vi "O2 Sensor Simulation.vi"(10 "Lambda":fxp<+,12,3>, 11 "Voltage at Ip in":fxp<+/-,16,5>) -> (0 "Ip":fxp<+/-,32,10>, 3 "Vn Out":fxp<+/-,20,5>)   [LabVIEW 2014]
uses:
  <vilib>/rvi/Analysis/measure/butterworth/XNode/niFpgaButterworthFilter.xnode
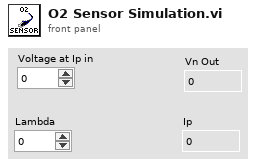
[diagram p1: front panel]
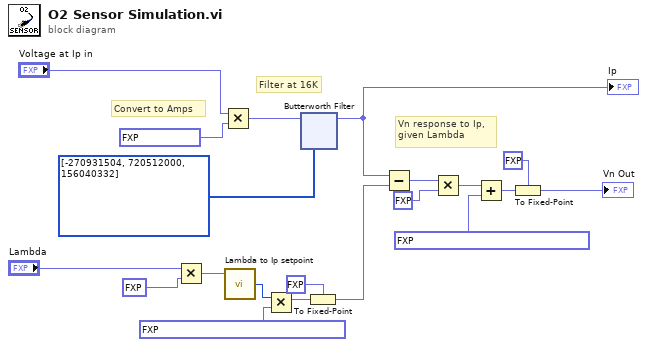
[diagram p0: block diagram]
diagram:
  # "Filter at 16K"
  # "Vn response to Ip, \ngiven Lambda"
  # "Convert to Amps"
  n1 = Multiply(x="Lambda", y=fxp<+,7,7> 100.0) -> (x*y=w17:fxp<+,19,10>)
  n2 = Multiply(x="Voltage at Ip in", y=fxp<+/-,16,5> 0.01611328125 ("V - A Scale Factor")) -> (x*y=w3:fxp<+/-,32,10>)
  n3 = call "Lambda to Ip setpoint"("address"=w17) -> ("data out"=w13:i16)  [unwired: 8 in]
  n4 = Multiply(x=w13, y=fxp<+,30,-4> 1.0000017937272787e-05) -> (x*y=w18:fxp<+/-,46,12>)
  n5 = xnode "Butterworth Filter"("input data"=w3, "scaled coefficients"=i32[] [-270931504, 720512000, 156040332]) -> ("output data"=w2:fxp<+/-,32,10>)  [unwired: 1 in]
  "Ip" <- w2
  n6 = To Fixed-Point(fixed-point type=fxp<+/-,20,5> 0.0 ("Ip setpoint"), number=w18) -> (fixed-point=w20:fxp<+/-,20,5>)
  n7 = Subtract(x=w2, y=w20) -> (x-y=w6:fxp<+/-,33,11>)
  n8 = Multiply(x=w6, y=fxp<+/-,21,8> 75.0 ("gain")) -> (x*y=w8:fxp<+/-,53,18>)
  n9 = Add(x=w8, y=fxp<+/-,41,11> 0.4500000001862645) -> (x+y=w10:fxp<+/-,53,18>)
  n10 = To Fixed-Point(fixed-point type=fxp<+/-,20,5> 0.0 ("Mod3/AO0"), number=w10) -> (fixed-point=→"Vn Out":fxp<+/-,20,5>)
